vi "Traffic Light with Arduino.vi"(4 "stop":bool) -> (0 "GREEN":bool, 1 "YELLOW":bool, 2 "RED":bool)   [LabVIEW 2015]
uses:
  <vilib>/MakerHub/LINX/Public/Peripherals/Digital/Digital Write N Chans.vi
  <vilib>/MakerHub/LINX/Private/Local IO/LinxDigitalWrite.vi
  <vilib>/MakerHub/LINX/Public/Utilities/Check Channel.vi
  <vilib>/MakerHub/LINX/Public/Utilities/Open Serial.vi
  <vilib>/MakerHub/LINX/Private/Utilties/Generate Error.vi
  <vilib>/MakerHub/LINX/LMH-LINX.lvlib
panel:
  in  "Serial Port":refnum<visa-resource-name>="N/A"
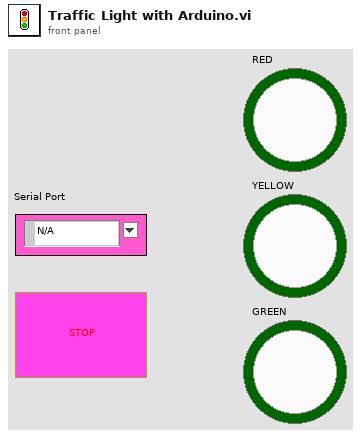
[diagram p1: front panel]
types:
  T1 = typedef "LMH-LINX.lvlib/LINX Ref.ctl" = cluster{"IO":T2, "Interface":T3, "LINX Device Config":T4}
  T2 = typedef "LMH-LINX.lvlib/Platform.ctl" = enum16{"Remote", "Local"}
  T3 = typedef "LMH-LINX.lvlib/Interface.ctl" = enum16{"Serial", "TCP"}
  T4 = typedef "LMH-LINX.lvlib/Device.lvlib/LINX Device Config.ctl" = cluster{"Interface":T3, "COM Port":refnum<visa-resource-name>, "TCP Configuration":T5, "Device Family":u8, "Device ID":u8, "Device Name":string, "TCP Ref":refnum<k5>, "Channels":T6}
  T5 = typedef "LMH-LINX.lvlib/Device.lvlib/TCP Config.ctl" = cluster{"IP Address":string, "Port":u16}
  T6 = typedef "LMH-LINX.lvlib/Channels.ctl" = cluster{"DI":u8[], "DO":u8[], "AI":u8[], "AO":u8[], "PWM":u8[], "QE":u8[], "UART":u8[], "I2C 2":u8[], "SPI":u8[], "CAN":u8[], "Servo":u8[], "AI Ref (V)":dbl, "AI Resolution (Bits)":u8, "AO Ref (V)":dbl, "AO Resolution (Bits)":u8}
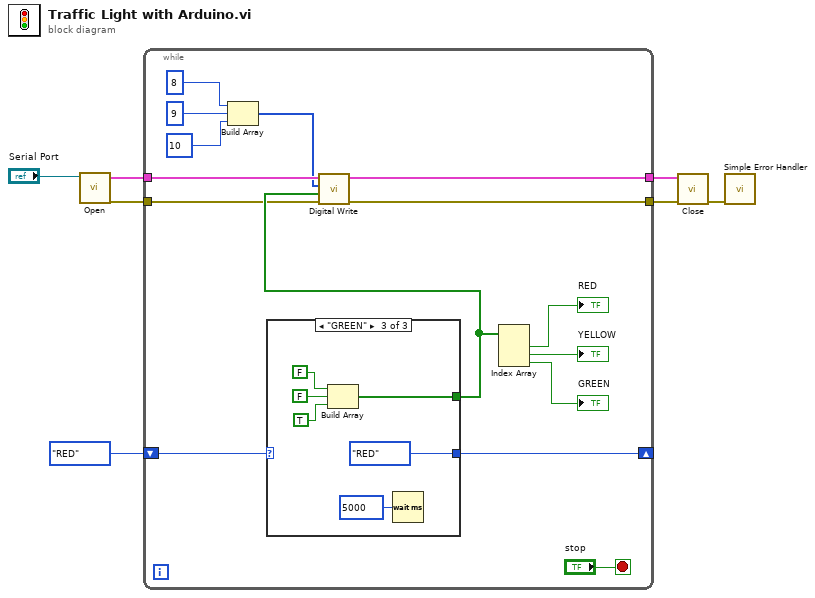
[diagram p0: block diagram]
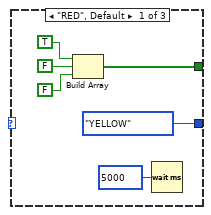
[diagram p2: hidden frame]
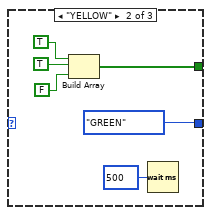
[diagram p3: hidden frame]
diagram:
  n1 = call-poly <vilib>:"Open.vi"("Serial Port"="Serial Port") -> ("Error Out"=w2:errorcluster, "LINX Resource"=w3:T1)  [unwired: 8 in, 1 out]
  n2 = while {
    shift-right: [w22] -> _
    shift-left: enum16{"RED", "YELLOW", "GREEN"}."RED" -> [w9]
    tunnel: w3 -> [w20]
    tunnel: [w15] -> w7
    tunnel: w2 -> [w14]
    tunnel: [w13] -> w6
    stop <- "stop" stop-if-true
    n3 = Build Array(8, 9, 10) -> (w17:i32[])
    n4 = case shown="\"GREEN\"" w9 {
      tunnel: [enum16{"RED", "YELLOW", "GREEN"}."YELLOW" enum16{"RED", "YELLOW", "GREEN"}."GREEN" enum16{"RED", "YELLOW", "GREEN"}."RED"] -> w22
      tunnel: [w28 w31 w37] -> w16
      frame "RED", Default {
        n5 = Build Array(TRUE, FALSE, FALSE) -> (w28:bool[])
        n6 = Wait (ms)(milliseconds to wait=u32 5000) -> ()  [unwired: 1 out]
      }
      frame "YELLOW" {
        n7 = Build Array(TRUE, TRUE, FALSE) -> (w31:bool[])
        n8 = Wait (ms)(milliseconds to wait=u32 500) -> ()  [unwired: 1 out]
      }
      frame "GREEN" {
        n9 = Build Array(FALSE, FALSE, TRUE) -> (w37:bool[])
        n10 = Wait (ms)(milliseconds to wait=u32 5000) -> ()  [unwired: 1 out]
      }
    }
    n11 = call-poly <vilib>:"Digital Write.vi"("Error In"=w14, "Values"=w16, "DO Channels"=w17, "LINX Resource"=w20) -> ("Error Out"=w13:errorcluster, "LINX Resource"=w15:T1)  [unwired: 6 in]
    n12 = Index Array(array=w16) -> (element #1=→"RED":bool, element #2=→"YELLOW":bool, element #3=→"GREEN":bool)  [unwired: 3 in]
  }
  n13 = call <vilib>:"Close.vi"("Error In"=w6, "LINX Resource"=w7) -> ("Error Out"=w5:errorcluster)  [unwired: 9 in]
  n14 = call <vilib>:"Simple Error Handler.vi"("error in (no error)"=w5) -> ()  [unwired: 4 in, 5 out]
